vi "zmien kierunek.vi"(11 "x":u8) -> (3 "x-y":u8)   [LabVIEW 2015]
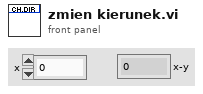
[diagram p1: front panel]
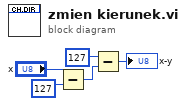
[diagram p0: block diagram]
diagram:
  n1 = Subtract(x="x", y=u8 127) -> (x-y=w1:u8)
  n2 = Subtract(x=u8 127, y=w1) -> (x-y=→"x-y":u8)
